vi "Simple Error Handler.vi"(3 "error code (no error:0)":i32 format="%0.0f", 4 "error source (\" \")":string, 8 "type of dialog (OK msg:1)":T1=1 items=["no dialog", "OK message", "continue or stop message", "OK message + warnings", "continue/stop + warnings"], 9 "error in (no error)":errorcluster) -> (0 "error?":bool, 1 "code out":i32 format="%0.0f", 5 "source out":string, 6 "error out":errorcluster, 7 "message":string=" INSTRUCTIONS:\r\rNormal Use:  When using subVIs that incorporate the error in/error out (or error I/O) structure, place this handler where you want to inform the user of an error, typically at the end of the I/O data path, as the last action of the program.  If the error in error? is ERROR, the handler creates a message describing the error and its source.  If the type of dialog = 1 (default), the message is displayed to the user, who can only acknowedge it.  If the type = 2, the user can acknowledge the message or abort execution; aborting a program with active I/O is not recommended.  If the type = 0, no message is displayed; this is used to process the error programmatically, and the error out cluster elements are wired to individual terminals for that reason.  \r\rOther Use:\n\r\nlocal testing.  To test the error code of a subVI or function that does not have the error I/O structure, you can wire its error code and a source string to the local error code and error source inputs.  If error in error? indicates no error and error code is not equal to 0, the local code and source are substituted for the error in values, and error? is set TRUE (ERROR).")   [LabVIEW 2010]
doc: "Indicates whether an error occurred. If an error occurred, this VI returns a description of the error and optionally displays a dialog box."
uses:
  <vilib>/Utility/error.llb/DialogType.ctl
panel:
  # "reinitialize to default to display instructions"
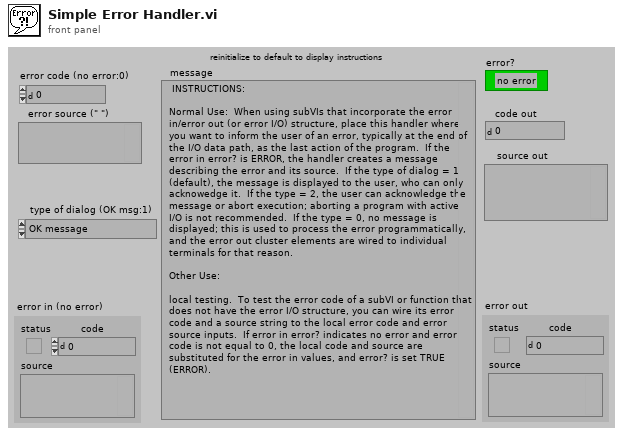
[diagram p1: front panel]
types:
  T1 = typedef "DialogType.ctl" = u16
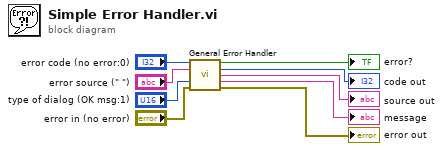
[diagram p0: block diagram]
diagram:
  n1 = call <vilib>:"General Error Handler.vi"("[error code] (0)"="error code (no error:0)", "[error source] (\" \")"="error source (\" \")", "type of dialog (OK msg:1)"="type of dialog (OK msg:1)", "error in (no error)"="error in (no error)") -> ("error?"=→"error?":bool, "code out"=→"code out":i32, "source out"=→"source out":string, "message"=→"message":string, "error out"=→"error out":errorcluster)  [unwired: 7 in]
